vi "Append Checksum.vi"(8 "error in":errorcluster, 10 "Message":u8[](array[numeric])) -> (0 "error out":errorcluster, 2 "Message w cksum":u8[](array[numeric]))   [LabVIEW 2019, in "ProXR.lvlib" / "ProXR.lvclass"]
uses:
  Library/ProXR.lvclass
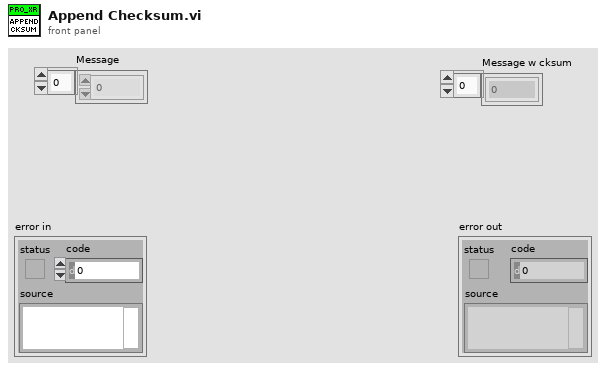
[diagram p1: front panel]
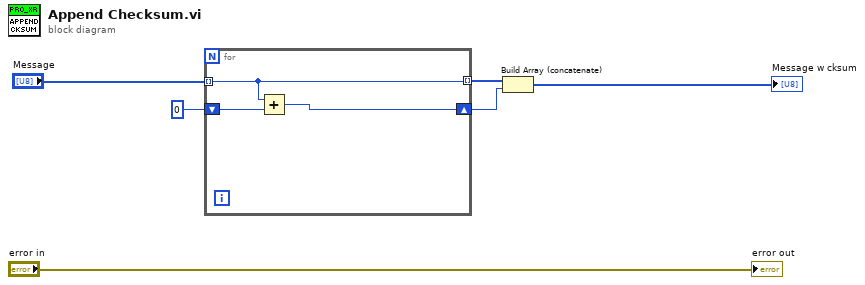
[diagram p0: block diagram]
diagram:
  n1 = for {
    tunnel: "Message" -> [w7] mode=indexing
    shift-right: [w8] -> w3
    shift-left: u8 0 ("Numeric") -> [w9]
    tunnel: [w7] -> w4 mode=indexing
    n2 = Add(x=w7, y=w9) -> (x+y=w8:u8)
  }
  n3 = Build Array (concatenate)(w4, w3) -> (→"Message w cksum":u8[])
  "error out" <- "error in"
